vi "Read Jitter Measurement (+Duty Cycle).vi"(8 "error in (no error)":errorcluster, 10 "Source +Duty Cycle (0: Channel 1)":u16(ring) items=["Channel 1", "Channel 2", "Channel 3", "Channel 4", "Math 1", "Math 2", "Math 3", "Math 4", "Reference Waveform 1", "Reference Waveform 2", "Reference Waveform 3", "Reference Waveform 4"], 11 "VISA resource name":refnum<visa-resource-name>) -> (0 "error out":errorcluster, 2 "+Duty Cycle":dbl, 3 "VISA resource name out":refnum<visa-resource-name>)   [LabVIEW 2015, in "Agilent 2000 3000 X-Series.lvlib"]
doc: "Returns a positive duty cycle measurement.\n\n<b>Note:</b>\nThis VI is specific to the 6000-X Series oscilloscopes. These features are not available on other models."
uses:
  <instrlib>/Agilent 2000 3000 X-Series/Agilent 2000 3000 X-Series.lvlib
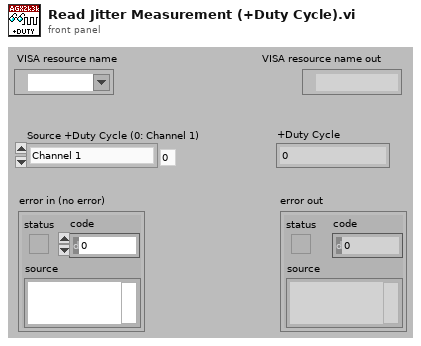
[diagram p1: front panel]
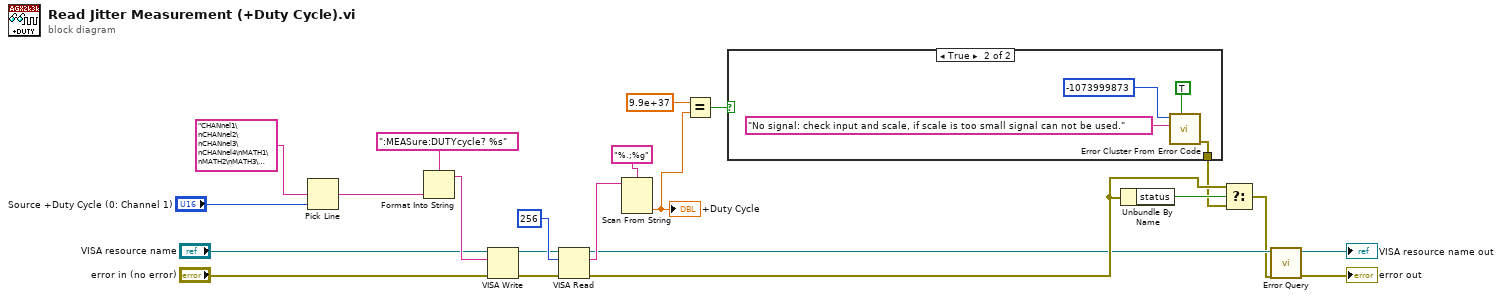
[diagram p0: block diagram]
diagram:
  n1 = Pick Line(multi-line string="CHANnel1\nCHANnel2\nCHANnel3\nCHANnel4\nMATH1\nMATH2\nMATH3\nMATH4\nWMEMory1\nWMEMory2\nWMEMory3\nWMEMory4", line index="Source +Duty Cycle (0: Channel 1)") -> (output string=w20:string)  [unwired: 1 in]
  n2 = Format Into String(format string=":MEASure:DUTYcycle? %s", w20) -> (resulting string=w19:string)  [unwired: 2 in, 1 out]
  n3 = VISA Write(VISA resource name="VISA resource name", write buffer=w19, error in (no error)="error in (no error)") -> (VISA resource name out=w3:refnum<visa-resource-name>, error out=w4:errorcluster)  [unwired: 1 out]
  n4 = VISA Read(VISA resource name=w3, byte count=u32 256, error in (no error)=w4) -> (VISA resource name out=w2:refnum<visa-resource-name>, read buffer=w13:string, error out=w7:errorcluster)  [unwired: 1 out]
  n5 = Scan From String(format string="%.;%g", input string=w13) -> (output 1=w9:dbl)  [unwired: 3 in, 3 out]
  "+Duty Cycle" <- w9
  n6 = Equal?(x=9.9e+37, y=w9) -> (x = y?=w11:bool)
  n7 = case shown="True" w11 {
    tunnel: [_ w23] -> w6
    frame False {
    }
    frame True {
      n8 = call <vilib>:"Error Cluster From Error Code.vi"("show call chain? (False)"=TRUE, "error message (\"\")"="No signal: check input and scale, if scale is too small signal can not be used." ("error message (\"\")"), "error code (0)"=-1073999873) -> ("error out"=w23:errorcluster)  [unwired: 6 in]
    }
  }
  n9 = Unbundle By Name(w7) -> ("status"=w8:bool)
  n10 = Select(t=w7, s=w8, f=w6) -> (s? t:f=w1:errorcluster)
  n11 = call <instrlib>:"Error Query.vi"("error in (no error)"=w1, "VISA resource name"=w2) -> ("error out"=→"error out":errorcluster, "VISA resource name out"=→"VISA resource name out":refnum<visa-resource-name>)  [unwired: 6 in, 2 out]
